vi "DN4_AI_ReadRawData32.vi"(0 "Task ID":u32, 2 "count":i32, 3 "error in (no error)":errorcluster) -> (7 "Task ID":u32, 8 "data":u32[](array[numeric]), 9 "start time":dbl, 10 "error out":errorcluster)   [LabVIEW 2009]
uses:
  Windows/System32/AdvLvDaq.dll
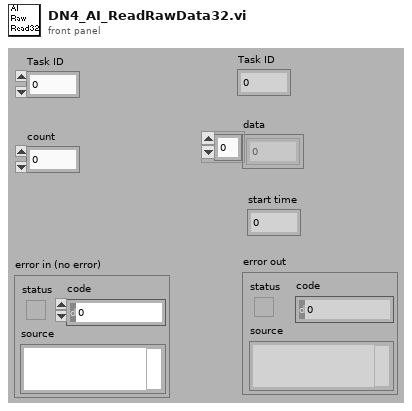
[diagram p1: front panel]
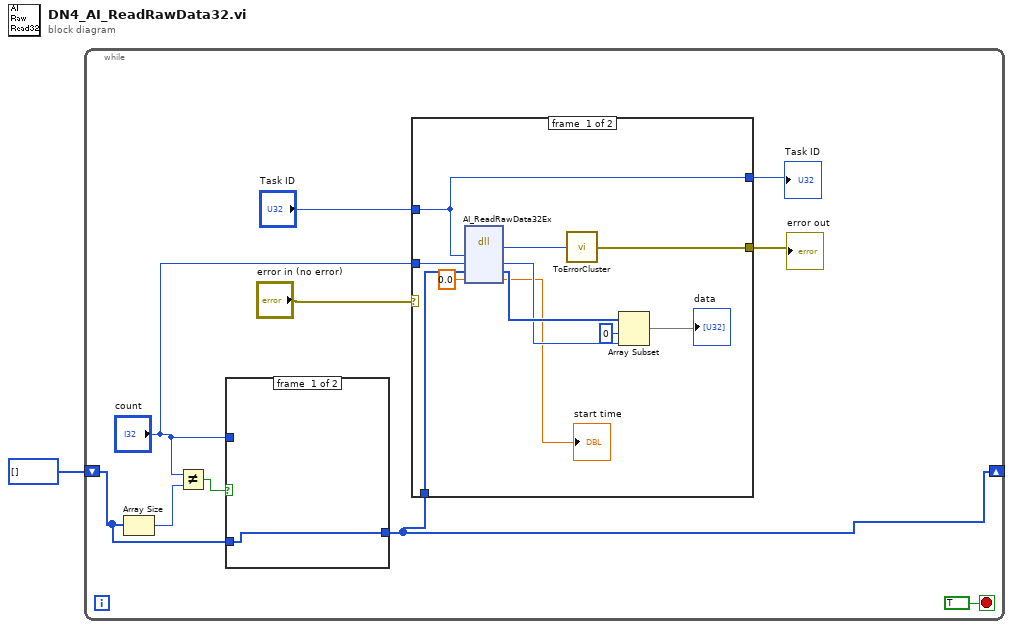
[diagram p0: block diagram]
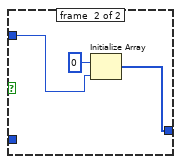
[diagram p2: hidden frame]
diagram:
  n1 = while {
    shift-right: [w2] -> _
    shift-left: u32[] [] -> [w4]
    stop <- TRUE stop-if-true
    n2 = Array Size(array=w4) -> (size(s)=w6:i32)
    n3 = Not Equal?(x="count", y=w6) -> (x != y?=w5:bool)
    n4 = case shown="True" w5 {
      tunnel: "count" -> [_ w14]
      tunnel: [w12 w13] -> w2
      tunnel: w4 -> [w12 _]
      frame #0 {
      }
      frame #1 {
        n5 = Initialize Array(u32 0 ("element"), w14) -> (w13:u32[])
      }
    }
    n6 = case shown="No Error" "error in (no error)" {
      selector: "error in (no error)" -> [_ w27]
      tunnel: "Task ID" -> [w24 w28]
      tunnel: [w25 w27] -> w9
      tunnel: [w24 w28] -> w8
      tunnel: "count" -> [w19 _]
      tunnel: w2 -> [w18 _]
      frame #0 {
        n7 = dll-call lib="C:/Windows/System32/AdvLvDaq.dll" fn="AI_ReadRawData32Ex"("taskId"=w24, "count"=w19, "data"=w18, "startTime"=0.0) -> ("return type"=w26:i32, "count"=w22:i32, "data"=w23:u32[], "startTime"=→"start time":dbl)  [unwired: 4 in, 2 out]
        n8 = call <userlib>:"ToErrorCluster.vi"("error code"=w26) -> ("error out"=w25:errorcluster)
        n9 = Array Subset(array=w23, index=0, length=w22) -> (→"data":u32[])
      }
      frame #1 {
      }
    }
    "error out" <- w9
    "Task ID" <- w8
  }
